vi "From CSV File.vi"(8 "error in (no error)":errorcluster, 9 "Path":path, 10 "engine in":refnum<class "engine configuration.lvclass">, 11 "Scan Engine editor node in":refnum<class "Scan Engine editor node.lvclass">) -> (0 "error out":errorcluster, 1 "Update":bool, 2 "engine out":refnum<class "engine configuration.lvclass">, 3 "Scan Engine editor node out":refnum<class "Scan Engine editor node.lvclass">)   [LabVIEW 2014, in "Scan Engine editor node.lvclass"]
uses:
  Scan Engine editor node.lvclass
  <vilib>/NI/Module Execution Interface/Engine Configuration/engine configuration.lvclass
  <vilib>/NI/DCAF/Tag Editor Core/Configuration Editor/Classes/Module editor node/module editor node.lvclass
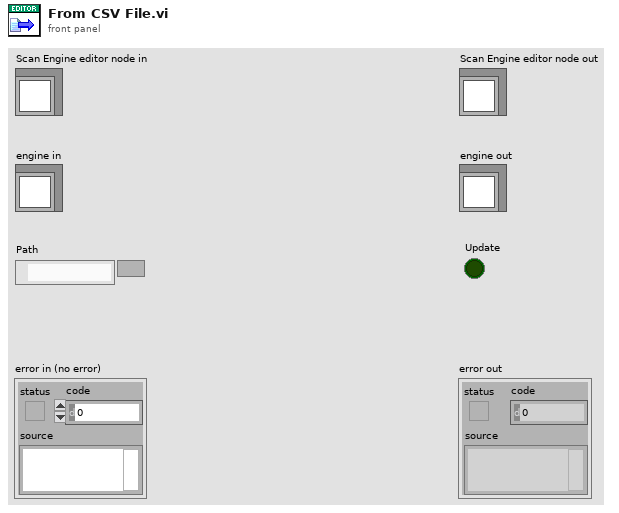
[diagram p1: front panel]
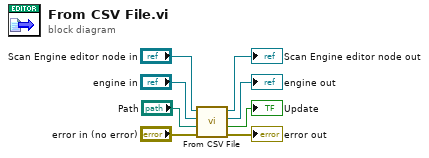
[diagram p0: block diagram]
diagram:
  n1 = call-parent "From CSV File.vi"("error in (no error)"="error in (no error)", "Path"="Path", "engine in"="engine in", "module editor node in"="Scan Engine editor node in") -> ("error out"=→"error out":errorcluster, "Update"=→"Update":bool, "engine out"=→"engine out":refnum<class "engine configuration.lvclass">, "module editor node out"=→"Scan Engine editor node out":refnum<class "Scan Engine editor node.lvclass">)  [unwired: 4 in]
